vi "Alignment_C.vi"(0 "Target":dbl format="%#_13g", 1 "Effort Addition":dbl=0.175 min=0.0 max=1.0 step=0.05 format="%#_13g", 2 "Camera Feedback":dbl=-79.93479492887602 format="%#_13g", 3 "Turn_Gain":dbl=0.25 format="%#_13g", 4 "Max Error":dbl=100.0 format="%#_13g", 5 "Range":dbl=32.301799999999986 format="%#_13g", 7 "POV":i32=180) -> (15 "Right Motor":dbl=-0.29408248732219006 format="%#_13g", 16 "Left Motor":dbl=0.29408248732219006 format="%#_13g", 17 "LeftAndRight?":bool)   [LabVIEW 2016]
panel:
  in  "LeftMotorSpeed":dbl format="%#_13g"
  in  "RightMotorSpeed":dbl format="%#_13g"
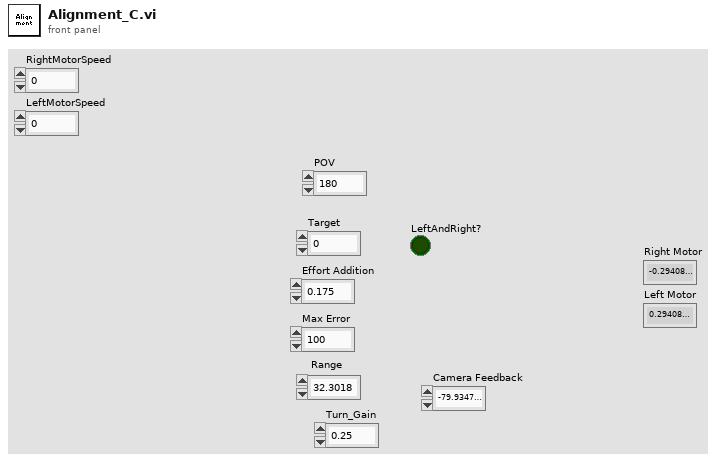
[diagram p1: front panel]
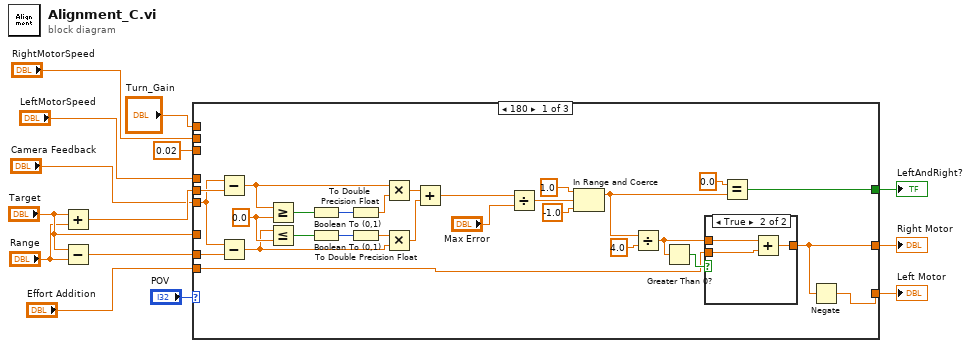
[diagram p0: block diagram]
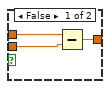
[diagram p2: hidden frame]
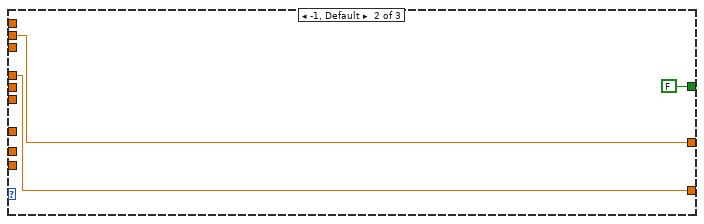
[diagram p3: hidden frame]
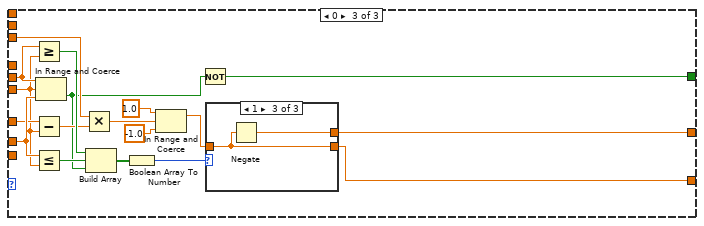
[diagram p4: hidden frame]
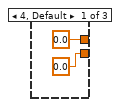
[diagram p5: hidden frame]
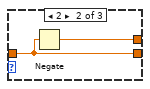
[diagram p6: hidden frame]
diagram:
  n1 = Add(x="Target", y="Range") -> (x+y=w7:dbl)
  n2 = Subtract(x="Target", y="Range") -> (x-y=w8:dbl)
  n3 = case shown="180" "POV" {
    tunnel: [w15 w51 w65] -> w1
    tunnel: "LeftMotorSpeed" -> [_ w51 _]
    tunnel: [w16 w50 w66] -> w3
    tunnel: "RightMotorSpeed" -> [_ w50 _]
    tunnel: "Camera Feedback" -> [w41 _ w60]
    tunnel: w7 -> [w42 _ w64]
    tunnel: w8 -> [w40 _ w69]
    tunnel: [w27 FALSE w52] -> w10
    tunnel: "Target" -> [_ _ w61]
    tunnel: 0.02 -> [_ _ w58]
    tunnel: "Turn_Gain" -> [_ _ _]
    tunnel: "Effort Addition" -> [w17 _ _]
    frame 180 {
      w39 = 0.0
      n4 = Subtract(x=w41, y=w42) -> (x-y=w37:dbl)
      n5 = Subtract(x=w41, y=w40) -> (x-y=w35:dbl)
      n6 = Greater Or Equal?(x=w37, y=w39) -> (x >= y?=w19:bool)
      n7 = Less Or Equal?(x=w35, y=w39) -> (x <= y?=w21:bool)
      n8 = Boolean To (0,1)(Boolean=w19) -> (0, 1=w18:i16)
      n9 = Boolean To (0,1)(Boolean=w21) -> (0, 1=w20:i16)
      n10 = To Double Precision Float(number=w18) -> (double precision float=w38:dbl)
      n11 = To Double Precision Float(number=w20) -> (double precision float=w36:dbl)
      n12 = Multiply(x=w37, y=w38) -> (x*y=w34:dbl)
      n13 = Multiply(x=w36, y=w35) -> (x*y=w33:dbl)
      n14 = Add(x=w34, y=w33) -> (x+y=w32:dbl)
      n15 = Divide(x=w32, y="Max Error") -> (x/y=w30:dbl)
      n16 = In Range and Coerce(upper limit=1.0, x=w30, lower limit=-1.0) -> (coerced(x)=w25:dbl)  [unwired: 1 out]
      n17 = Divide(x=w25, y=4.0) -> (x/y=w22:dbl)
      n18 = Greater Than 0?(x=w22) -> (x > 0?=w23:bool)
      n19 = case shown="True" w23 {
        tunnel: w22 -> [w45 w48]
        tunnel: [w44 w47] -> w16
        tunnel: w17 -> [w43 w46]
        frame False {
          n20 = Subtract(x=w45, y=w43) -> (x-y=w44:dbl)
        }
        frame True {
          n21 = Add(x=w48, y=w46) -> (x+y=w47:dbl)
        }
      }
      n22 = Equal?(x=0.0, y=w25) -> (x = y?=w27:bool)
      n23 = Negate(x=w16) -> (-x=w15:dbl)
    }
    frame -1, Default {
    }
    frame 0 {
      n24 = Greater Or Equal?(x=w64, y=w60) -> (x >= y?=w63:bool)
      n25 = Subtract(x=w61, y=w60) -> (x-y=w59:dbl)
      n26 = Less Or Equal?(x=w69, y=w60) -> (x <= y?=w62:bool)
      n27 = In Range and Coerce(upper limit=w64, x=w60, lower limit=w69) -> (In Range?=w53:bool)  [unwired: 1 out]
      n28 = Multiply(x=w58, y=w59) -> (x*y=w57:dbl)
      n29 = Build Array(w63, w62, w53) -> (w68:bool[])
      n30 = Boolean Array To Number(Boolean array=w68) -> (number=w67:u32)
      n31 = In Range and Coerce(upper limit=1.0, x=w57, lower limit=-1.0) -> (coerced(x)=w56:dbl)  [unwired: 1 out]
      n32 = Not(x=w53) -> (.not. x?=w52:bool)
      n33 = case shown="1" w67 {
        tunnel: [0.0 w72 w74] -> w66
        tunnel: [0.0 w73 w75] -> w65
        tunnel: w56 -> [_ w73 w75]
        frame 4, Default {
        }
        frame 2 {
          n34 = Negate(x=w73) -> (-x=w72:dbl)
        }
        frame 1 {
          n35 = Negate(x=w75) -> (-x=w74:dbl)
        }
      }
    }
  }
  "Left Motor" <- w1
  "Right Motor" <- w3
  "LeftAndRight?" <- w10
